vi "Read ASK File.vi"(8 "error in":errorcluster, 10 "Scan (T) / Median (F)":bool, 11 "File Path":path) -> (0 "error out":errorcluster, 3 "Data Cluster Out":T1)   [LabVIEW 2016]
uses:
  <vilib>/regexp/Match Regular Expression.xnode
panel:
  in  "Data Cluster":T1
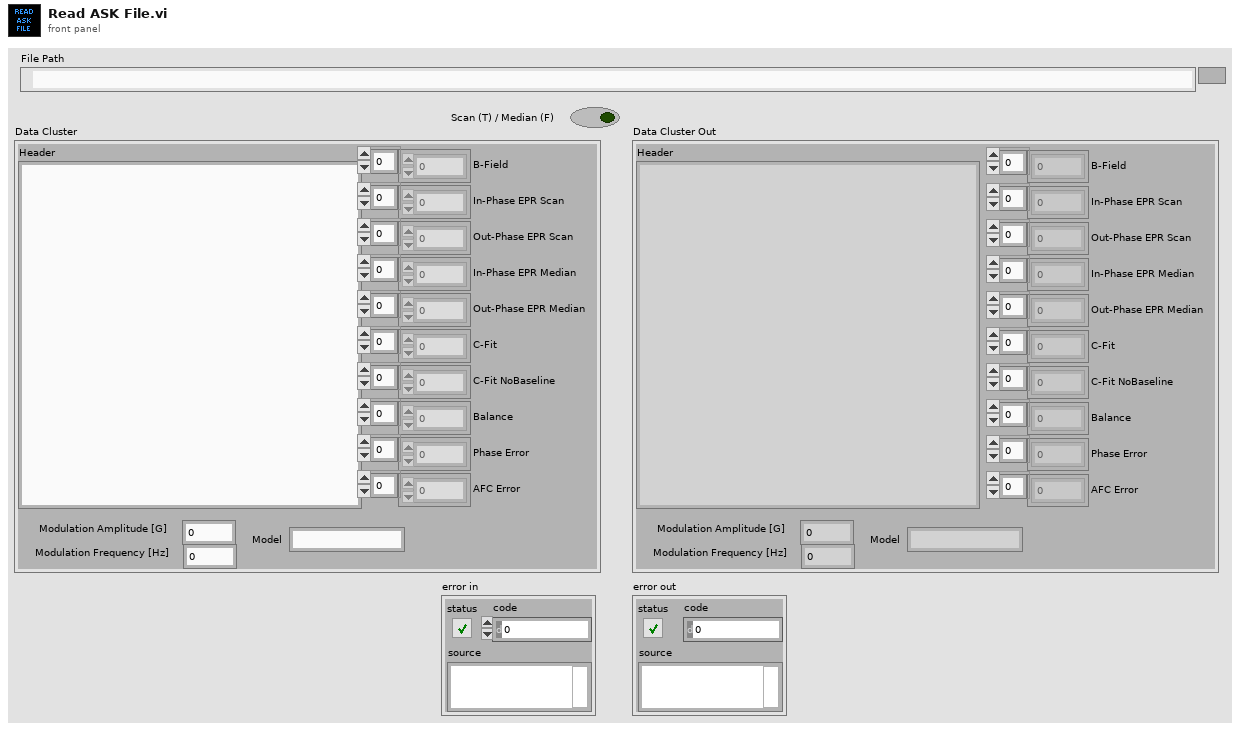
[diagram p1: front panel]
types:
  T1 = cluster{"Header":string, "B-Field":dbl[], "In-Phase EPR Scan":dbl[], "Out-Phase EPR Scan":dbl[], "Balance":dbl[], "Phase Error":dbl[], "AFC Error":dbl[], "Out-Phase EPR Median":dbl[], "In-Phase EPR Median":dbl[], "C-Fit":dbl[], "C-Fit NoBaseline":dbl[], "Modulation Amplitude [G]":dbl, "Modulation Frequency [Hz]":dbl, "Model":string}
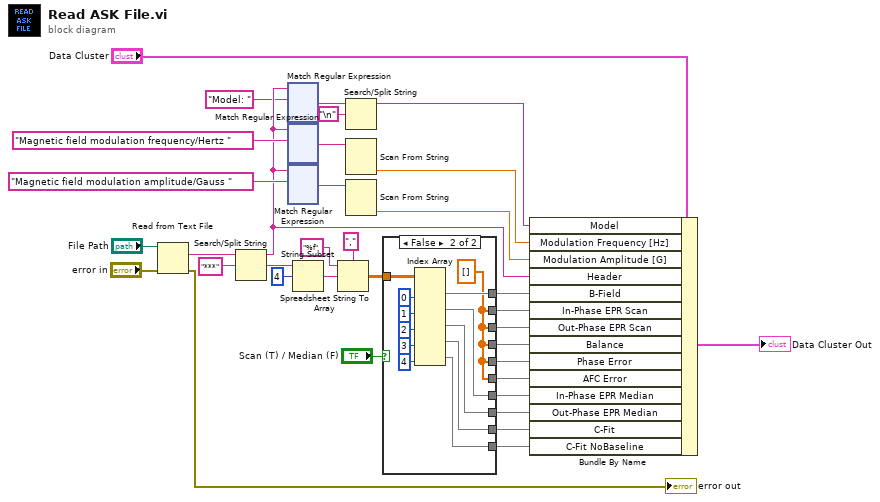
[diagram p0: block diagram]
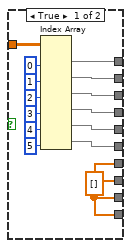
[diagram p2: hidden frame]
diagram:
  n1 = Read from Text File(file (use dialog)="File Path", error in="error in") -> (text=w34:string, error out=→"error out":errorcluster)  [unwired: 2 in, 2 out]
  n2 = Search/Split String(string=w34, search string/char (-)="***") -> (substring before match=w5:string, match + rest of string=w32:string)  [unwired: 1 in, 1 out]
  n3 = xnode "Match Regular Expression"("input string"=w5, "regular expression"="Model: ") -> ("after match"=w3:string)  [unwired: 4 in, 4 out]
  n4 = xnode "Match Regular Expression"("input string"=w5, "regular expression"="Magnetic field modulation frequency/Hertz " ("search string")) -> ("after match"=w10:string)  [unwired: 4 in, 4 out]
  n5 = xnode "Match Regular Expression"("input string"=w5, "regular expression"="Magnetic field modulation amplitude/Gauss " ("search string")) -> ("after match"=w8:string)  [unwired: 4 in, 4 out]
  n6 = String Subset(string=w32, offset (0)=4) -> (substring=w30:string)  [unwired: 1 in]
  n7 = Spreadsheet String To Array(delimiter (Tab)=",", format string="%f", spreadsheet string=w30) -> (array=w27:dbl[][])  [unwired: 1 in]
  n8 = Search/Split String(string=w3, search string/char (-)="\n") -> (substring before match=w1:string)  [unwired: 1 in, 2 out]
  n9 = Scan From String(input string=w10) -> (output 1=w6:dbl)  [unwired: 4 in, 3 out]
  n10 = Scan From String(input string=w8) -> (output 1=w7:dbl)  [unwired: 4 in, 3 out]
  n11 = case shown="False" "Scan (T) / Median (F)" {
    tunnel: w27 -> [w49 w61]
    tunnel: [w42 w55] -> w24
    tunnel: [w41 w50] -> w23
    tunnel: [w40 w50] -> w22
    tunnel: [w39 w50] -> w21
    tunnel: [w38 w50] -> w20
    tunnel: [w37 w50] -> w19
    tunnel: [w36 w54] -> w18
    tunnel: [w36 w53] -> w17
    tunnel: [w36 w52] -> w16
    tunnel: [w36 w51] -> w15
    frame True {
      w36 = dbl[] []
      n12 = Index Array(array=w49, index (col) #1=0 ("disabled index (col)"), index (col) #2=1 ("index (col)"), index (col) #3=2 ("index (col)"), index (col) #4=3 ("index (col)"), index (col) #5=4 ("index (col)"), index (col) #6=5 ("index (col)")) -> (element #1=w42:dbl[], element #2=w41:dbl[], element #3=w40:dbl[], element #4=w39:dbl[], element #5=w38:dbl[], element #6=w37:dbl[])  [unwired: 6 in]
    }
    frame False {
      w50 = dbl[] []
      n13 = Index Array(array=w61, index (col) #1=0 ("disabled index (col)"), index (col) #2=1 ("index (col)"), index (col) #3=2 ("index (col)"), index (col) #4=3 ("index (col)"), index (col) #5=4 ("index (col)")) -> (element #1=w55:dbl[], element #2=w54:dbl[], element #3=w53:dbl[], element #4=w52:dbl[], element #5=w51:dbl[])  [unwired: 5 in]
    }
  }
  n14 = Bundle By Name(cluster="Data Cluster", "Model"=w1, "Modulation Frequency [Hz]"=w6, "Modulation Amplitude [G]"=w7, "Header"=w5, "B-Field"=w24, "In-Phase EPR Scan"=w23, "Out-Phase EPR Scan"=w22, "Balance"=w21, "Phase Error"=w20, "AFC Error"=w19, "In-Phase EPR Median"=w18, "Out-Phase EPR Median"=w17, "C-Fit"=w16, "C-Fit NoBaseline"=w15) -> (→"Data Cluster Out":T1)
